vi "Add file to dependencie.vi"(7 "ForceDownload?(F)":bool, 9 "SupportedTarget":T1=enum."Linux_x64", 10 "RT Destination folder (c:\\ni-rt\\NIVeriStand)":path=path "c:/ni-rt/NIVeriStand", 11 "item path":path) -> (2 "destination path":path, 3 "dependency out":T2={"Source"={"Path"=path "", "Type"=enum."Absolute"}, "RT Destination"=path "", "ForceDownload?"=FALSE, "SupportedTarget"=enum."PharLap", "Version"=""})   [LabVIEW 2019, in "HLA Custom Device System Explorer.lvlib"]
uses:
  HLA Custom Device System Explorer.lvlib
  <vilib>/NI VeriStand/Custom Device API/Custom Device File Dependency.ctl
  <vilib>/NI VeriStand/Custom Device API/Path Specification.ctl
  <vilib>/NI VeriStand/Custom Device API/Path Type.ctl
  <vilib>/NI VeriStand/Custom Device API/Custom Device Supported Target.ctl
  <vilib>/NI VeriStand/Custom Device API/Custom Device API.lvlib
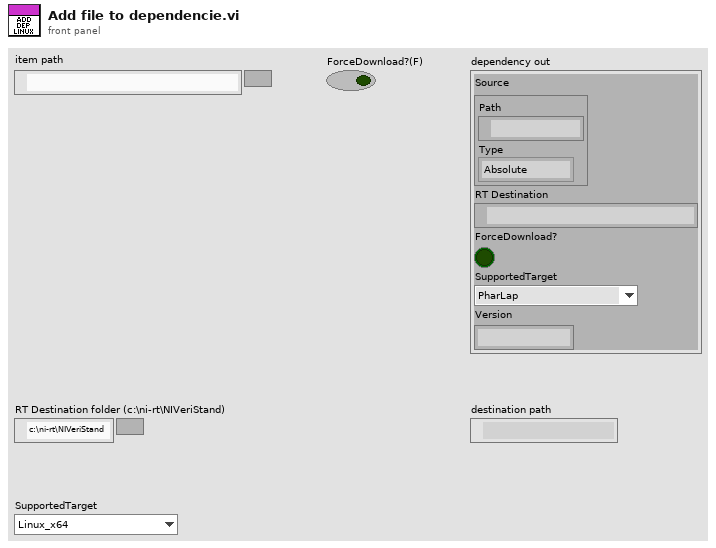
[diagram p1: front panel]
types:
  T1 = typedef "Custom Device API.lvlib/Custom Device Supported Target.ctl" = enum16{"All", "PharLap", "VxWorks", "Windows", "Linux_32_ARM", "Linux_x64", "PharLap & Windows", "PharLap & VxWorks", "VxWorks & Windows"}
  T2 = typedef "Custom Device API.lvlib/Custom Device File Dependency.ctl" = cluster{"Source":T3, "RT Destination":path, "ForceDownload?":bool, "SupportedTarget":T1, "Version":string}
  T3 = typedef "Custom Device API.lvlib/Path Specification.ctl" = cluster{"Path":path, "Type":T4}
  T4 = typedef "Custom Device API.lvlib/Path Type.ctl" = enum16{"Absolute", "To Base", "To Common Data Dir", "To Application Data Dir"}
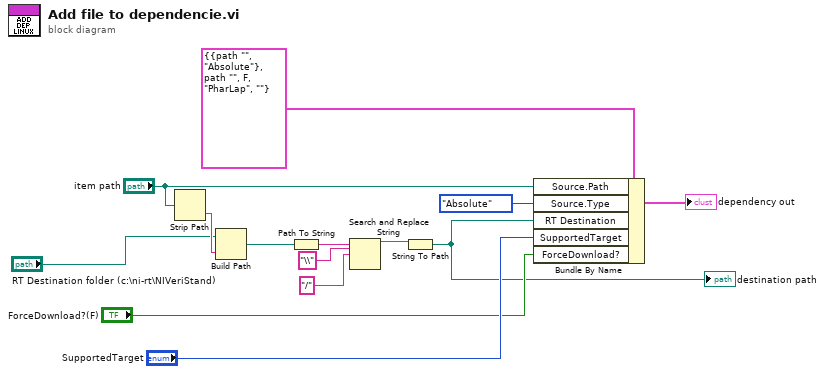
[diagram p0: block diagram]
diagram:
  n1 = Strip Path(path="item path") -> (name=w9:string)  [unwired: 1 out]
  n2 = Build Path(base path="RT Destination folder (c:\\ni-rt\\NIVeriStand)", name or relative path=w9) -> (appended path=w7:path)
  n3 = Path To String(path=w7) -> (string=w3:string)
  n4 = Search and Replace String(input string=w3, search string="\\", replace string="/" ("search string")) -> (result string=w4:string)  [unwired: 5 in, 3 out]
  n5 = String To Path(string=w4) -> (path=w5:path)
  "destination path" <- w5
  n6 = Bundle By Name(cluster=T2 {"Source"={"Path"=path "", "Type"=enum."Absolute"}, "RT Destination"=path "", "ForceDownload?"=FALSE, "SupportedTarget"=enum."PharLap", "Version"=""} ("Dependencies"), "Source.Path"="item path", "Source.Type"=Path_Type."Absolute", "RT Destination"=w5, "SupportedTarget"="SupportedTarget", "ForceDownload?"="ForceDownload?(F)") -> (→"dependency out":T2)
